vi "Sleep.vi"() -> (0 "Wokeup":bool)   [LabVIEW 2024]
doc: "The VI hanged until the notifier \"Wakeup\" is activated."
uses:
  Globals and TypeDefs/gStatus.vi
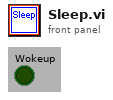
[diagram p1: front panel]
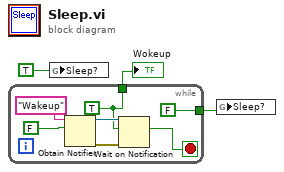
[diagram p0: block diagram]
diagram:
  n1 = while {
    tunnel: [w5] -> w3
    tunnel: [FALSE ("Sleep?")] -> w1
    stop <- w6 stop-if-true
    w5 = TRUE ("ignore previous (F)")
    n2 = Obtain Notifier(name (unnamed)="Wakeup", notification data type=FALSE ("Auto Reset")) -> (notifier out=w8:refnum<notifier>, error out=w7:errorcluster)  [unwired: 2 in, 1 out]
    n3 = Wait on Notification(notifier=w8, ignore previous (F)=w5, error in (no error)=w7) -> (notification=w6:bool)  [unwired: 1 in, 3 out]
  }
  "Wokeup" <- w3
  n4 = global write "gStatus.vi" "Sleep?"(TRUE ("Sleep?")) -> ()
  n5 = global write "gStatus.vi" "Sleep?"(w1) -> ()
